vi "TestWaveformGeneration.vi"() -> ()   [LabVIEW 2015]
uses:
  Tek shared libraries/ArbitraryFunctions.lvlib
panel:
  out "sample rate (Hz)":dbl
  out "High Frequency OUT":dbl=100000.0
  out "Low Frequency OUT":dbl=100000.0
  in  "Low Frequ. Harmonic":dbl=1.0 format="%#_13g"
  out "Waveform Graph":dbl[](graph)
  in  "Probe Frequency":dbl=86000000.0
  in  "WaveDuration (us)":dbl=2e-05
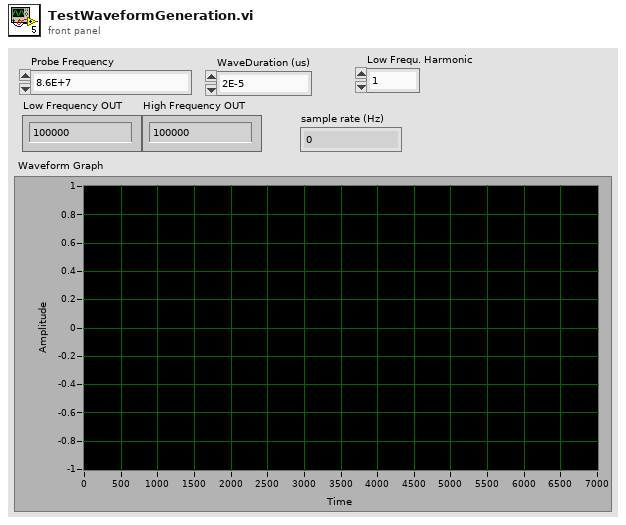
[diagram p1: front panel]
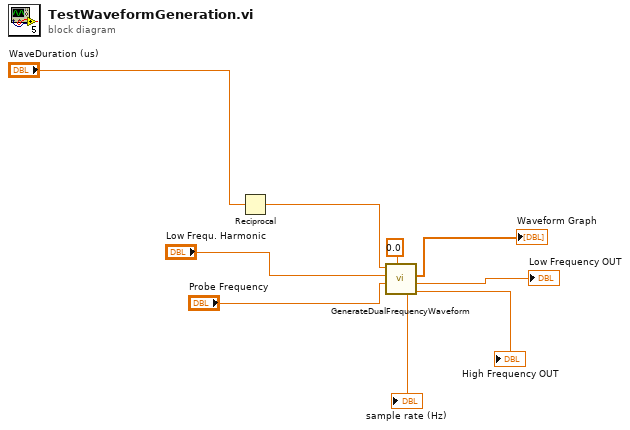
[diagram p0: block diagram]
diagram:
  n1 = Reciprocal(x="WaveDuration (us)") -> (1/x=w6:dbl)
  n2 = call "GenerateDualFrequencyWaveform.vi"("Phase (2pi unit)"=0.0, "High Frequency IN"="Probe Frequency", "Harmonic"="Low Frequ. Harmonic", "Low Frequency IN"=w6) -> ("High Frequency OUT"=→"High Frequency OUT":dbl, "Low Frequency OUT"=→"Low Frequency OUT":dbl, "Waveform Graph"=→"Waveform Graph":dbl[], "sample rate (Hz)"=→"sample rate (Hz)":dbl)  [unwired: 3 in, 1 out]
